vi "Set Error Handler.vi"(8 "error in (no error)":errorcluster, 10 "Error Handler":refnum<class "Error Handler Interface.lvclass">, 11 "Process In":refnum<class "Process.lvclass">) -> (0 "error out":errorcluster, 3 "Process Out":refnum<class "Process.lvclass">)   [LabVIEW 2020, in "Process.lvclass"]
doc: "Set the error handler for the process. The error handler Handle Errors.vi interface is then called by the Handle Process Errors.vi method."
uses:
  Process.lvclass
  Error Handler Interface/Error Handler Interface.lvclass
  Process.lvclass/Process.ctl
  Private/SubVIs/Handle Debug Data.vi
  Logging/Log Debug.vi
  <vilib>/AdvancedString/1D String Array to Delimited String.vi
  <vilib>/Utility/High Resolution Relative Seconds.vi
  <vilib>/Utility/error.llb/Error Cluster From Error Code.vi
  Read Name.vi
  Callback/Callback.lvclass
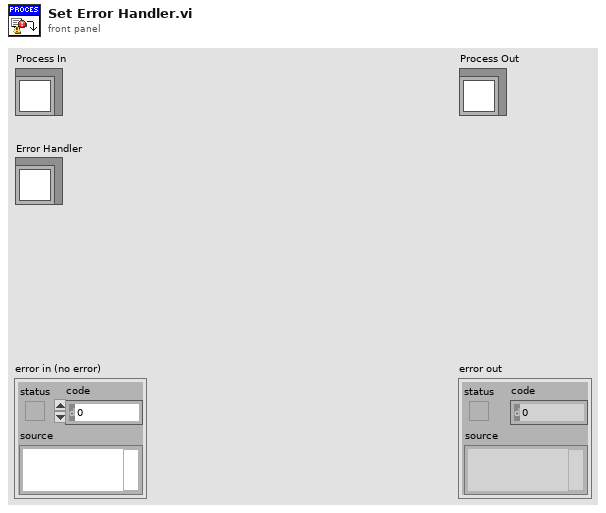
[diagram p1: front panel]
types:
  T1 = typedef "Process.lvclass/API Mode.ctl" = enum16{"Send Message", "Handle Message"}
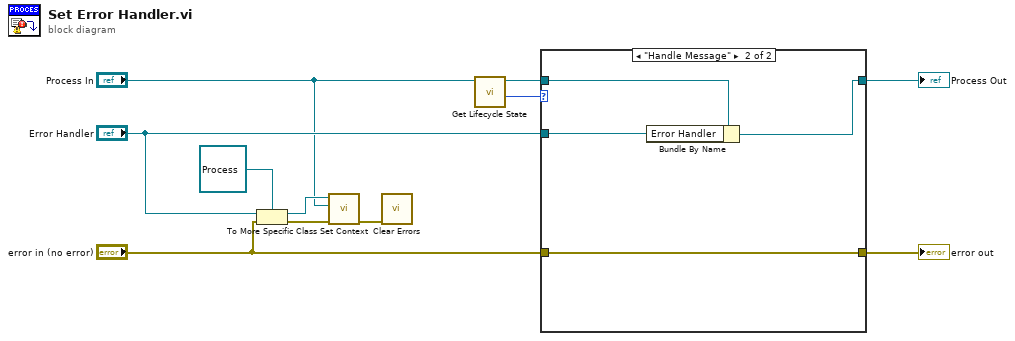
[diagram p0: block diagram]
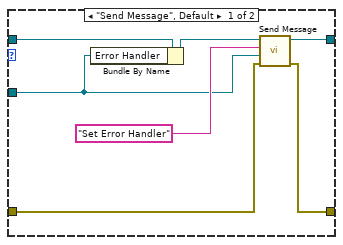
[diagram p2: hidden frame]
diagram:
  n1 = To More Specific Class(target class=refnum<class "Process.lvclass"> refnum ("Process In"), reference="Error Handler", error in="error in (no error)") -> (specific class reference=w7:refnum<class "Process.lvclass">, error out=w4:errorcluster)
  n2 = call "Set Context.vi"("error in (no error)"=w4, "Process Context"="Process In", "Process In"=w7) -> ("error out"=w2:errorcluster)  [unwired: 7 in, 1 out]
  n3 = call <vilib>:"Clear Errors.vi"("error in (no error)"=w2) -> ()  [unwired: 5 in, 2 out]
  n4 = call "Get Lifecycle State.vi"("Process In"="Process In") -> ("API Mode"=w10:T1, "Process Out"=w11:refnum<class "Process.lvclass">)  [unwired: 7 in, 2 out]
  n5 = case shown="\"Handle Message\"" w10 {
    tunnel: w11 -> [w18 w22]
    tunnel: [w17 w19] -> w8
    tunnel: "error in (no error)" -> [w15 w20]
    tunnel: [w16 w20] -> w9
    tunnel: "Error Handler" -> [w12 w21]
    frame "Send Message", Default {
      n6 = Bundle By Name(cluster=w18, "Error Handler"=w12) -> (w13:refnum<class "Process.lvclass">)
      n7 = call "Send Message.vi"("error in (no error)"=w15, "Message Data"=w12, "Message"="Set Error Handler", "Process In"=w13) -> ("error out"=w16:errorcluster, "Process Out"=w17:refnum<class "Process.lvclass">)  [unwired: 6 in]
    }
    frame "Handle Message" {
      n8 = Bundle By Name(cluster=w22, "Error Handler"=w21) -> (w19:refnum<class "Process.lvclass">)
    }
  }
  "error out" <- w9
  "Process Out" <- w8
